vi "cam0-镜像槽点对应中心槽角计算.vi"(9 "位置参数":T1={"槽点位"={"X"=125.0, "Y"=75.0}, "产品位"={"X"=150.0, "Y"=100.0}, "各槽角"=[], "中心位"={"X"=100.0, "Y"=100.0}, "中心产品半径"=0.0, "最接近槽角序号"=0, "槽在中心到产品连线所在侧"=enum."左侧-逆时针向", "中心位到产品位指向角"=0.0}) -> (0 "匹配槽OK":bool, 2 "匹配到的槽角序号":i32, 3 "槽点偏距与产品半径比":dbl format="%.2f")   [LabVIEW 2018]
uses:
  <vilib>/vision/NI_Vision_Development_Module.lvlib
panel:
  # "槽点偏距与产品半径比，表示槽的对正程度，用于确定是否可以将该槽用于铜碎检测"
  # "反映了槽偏离中心线的程度"
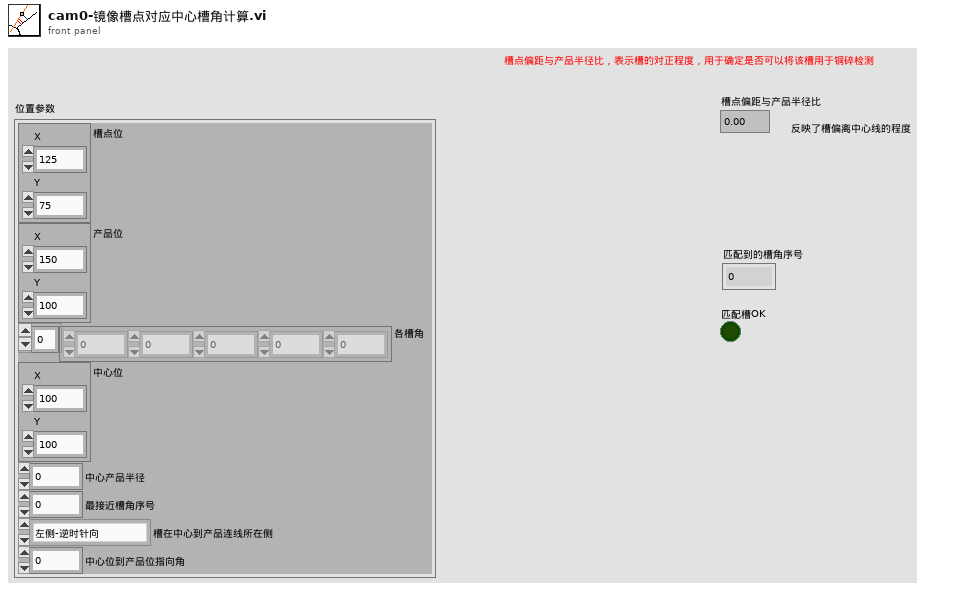
[diagram p1: front panel]
types:
  T1 = cluster{"槽点位":cluster{"X":sgl, "Y":sgl}, "产品位":cluster{"X":sgl, "Y":sgl}, "各槽角":dbl[], "中心位":cluster{"X":sgl, "Y":sgl}, "中心产品半径":sgl, "最接近槽角序号":i32, "槽在中心到产品连线所在侧":enum16{"左侧-逆时针向", "右侧-顺时针向"}, "中心位到产品位指向角":sgl}
  T2 = cluster{"产品位":cluster{"X":sgl, "Y":sgl}, "中心位":cluster{"X":sgl, "Y":sgl}}
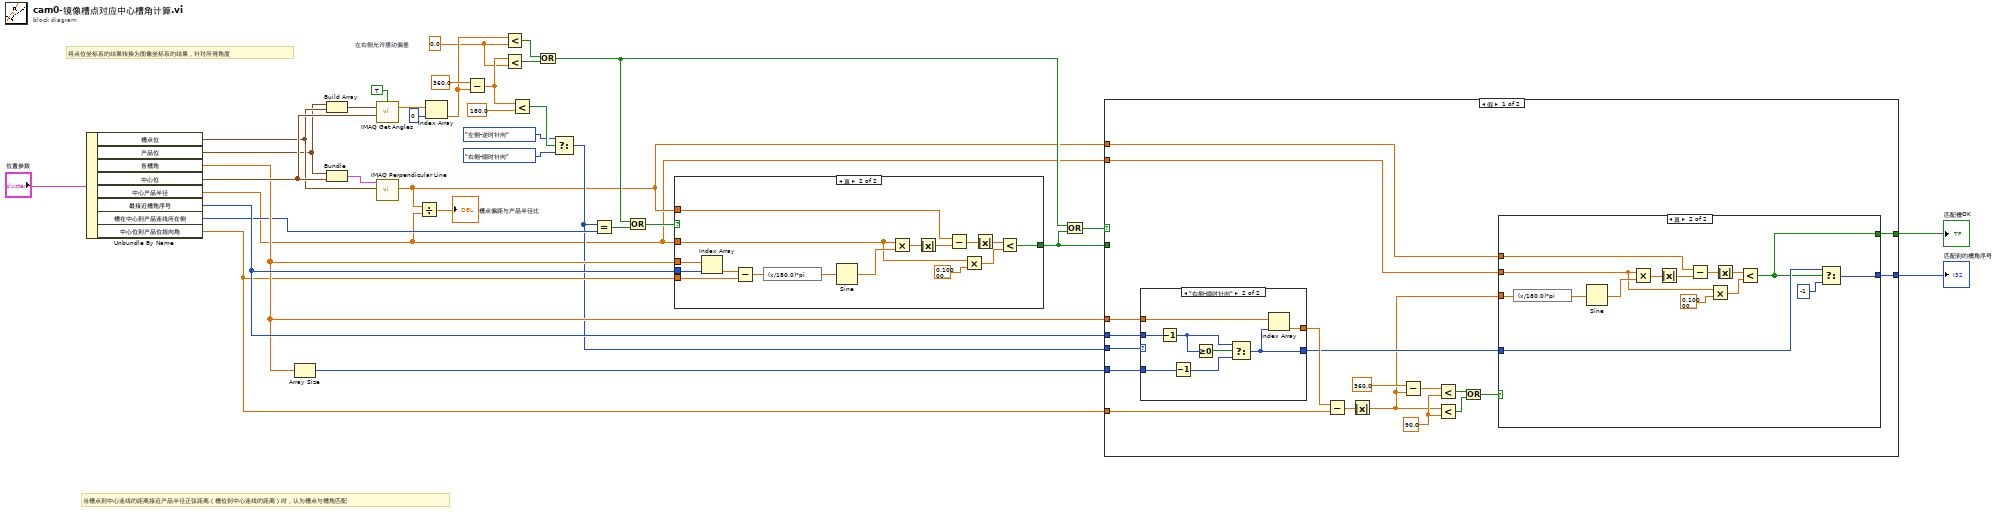
[diagram p0: block diagram]
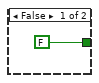
[diagram p2: hidden frame]
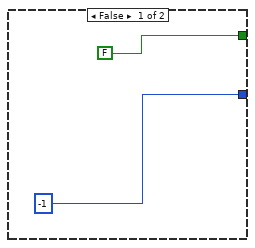
[diagram p3: hidden frame]
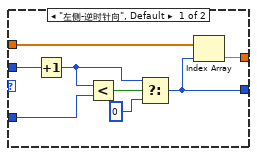
[diagram p4: hidden frame]
diagram:
  w11 = sgl 0.0  # 左右侧允许摆动偏差
  # "当槽点到中心连线的距离接近产品半径正弦距离（槽位到中心连线的距离）时，认为槽点与槽角匹配"
  # "将点位坐标系的结果转换为图像坐标系的结果，针对所得角度"
  n1 = Unbundle By Name("位置参数") -> ("槽点位"=w27:cluster{"X":sgl, "Y":sgl}, "产品位"=w26:cluster{"X":sgl, "Y":sgl}, "各槽角"=w22:dbl[], "中心位"=w28:cluster{"X":sgl, "Y":sgl}, "中心产品半径"=w2:sgl, "最接近槽角序号"=w24:i32, "槽在中心到产品连线所在侧"=w15:enum16{"左侧-逆时针向", "右侧-顺时针向"}, "中心位到产品位指向角"=w21:sgl)
  n2 = Array Size(array=w22) -> (size(s)=w23:i32)
  n3 = Build Array(w26, w27) -> (w31:cluster{"X":sgl, "Y":sgl}[])
  n4 = Bundle("产品位"=w26, "中心位"=w28) -> (w35:T2)  [unwired: 1 in]
  n5 = call "IMAQ Get Angles"("Vertex"=w28, "Points"=w31, "Use Vertex (No)"=TRUE) -> ("Angles (deg)"=w33:sgl[])  [unwired: 2 in, 2 out]
  n6 = call "IMAQ Perpendicular Line"("Point"=w27, "Line"=w35) -> ("Distance"=w3:dbl)  [unwired: 7 in, 2 out]
  n7 = Divide(x=w3, y=w2) -> (x/y=→"槽点偏距与产品半径比":dbl)
  n8 = Index Array(array=w33, index=0 ("索引")) -> (element=w12:sgl)
  n9 = Subtract(x=sgl 360.0, y=w12) -> (x-y=w13:sgl)
  n10 = Less?(x=w12, y=w11) -> (x < y?=w9:bool)
  n11 = Less?(x=w13, y=w11) -> (x < y?=w10:bool)
  n12 = Less?(x=w13, y=sgl 180.0) -> (x < y?=w18:bool)
  n13 = Or(x=w9, y=w10) -> (x .or. y?=w6:bool)
  n14 = Select(t=enum16{"左侧-逆时针向", "右侧-顺时针向"}."左侧-逆时针向" ("槽在中心到产品连线所在侧"), s=w18, f=enum16{"左侧-逆时针向", "右侧-顺时针向"}."右侧-顺时针向" ("槽在中心到产品连线所在侧")) -> (s? t:f=w14:enum16{"左侧-逆时针向", "右侧-顺时针向"})
  n15 = Equal?(x=w14, y=w15) -> (x = y?=w4:bool)
  n16 = Or(x=w6, y=w4) -> (x .or. y?=w5:bool)
  n17 = case shown="真" w5 {
    tunnel: [FALSE w44] -> w7
    tunnel: w24 -> [_ w43]
    tunnel: w22 -> [_ w42]
    tunnel: w21 -> [_ w41]
    tunnel: w3 -> [_ w39]
    tunnel: w2 -> [_ w37]
    frame False {
    }
    frame True {
      n18 = Index Array(array=w42, index=w43) -> (element=w45:dbl)
      n19 = Subtract(x=w45, y=w41) -> (x-y=w40:dbl)
      n20 = expression code="(x/180.0)*pi" ("degrees to radians")(w40) -> (w52:dbl)
      n21 = Sine(x=w52) -> (sin(x)=w51:dbl)
      n22 = Multiply(x=w37, y=w51) -> (x*y=w50:dbl)
      n23 = Absolute Value(x=w50) -> (abs(x)=w49:dbl)
      n24 = Subtract(x=w39, y=w49) -> (x-y=w48:dbl)
      n25 = Multiply(x=w37, y=sgl 0.1) -> (x*y=w38:sgl)
      n26 = Absolute Value(x=w48) -> (abs(x)=w47:dbl)
      n27 = Less?(x=w47, y=w38) -> (x < y?=w44:bool)
    }
  }
  n28 = Or(x=w6, y=w7) -> (x .or. y?=w8:bool)
  n29 = case shown="假" w8 {
    tunnel: [w57 w105] -> w25
    tunnel: w24 -> [w70 w106]
    tunnel: w14 -> [w71 _]
    tunnel: w23 -> [w69 _]
    tunnel: w22 -> [w68 _]
    tunnel: w21 -> [w66 _]
    tunnel: w3 -> [w56 _]
    tunnel: [w58 w106] -> w20
    tunnel: w2 -> [w55 _]
    tunnel: w7 -> [_ w105]
    frame False {
      w63 = 90.0 ("y")
      n30 = case shown="\"右侧-顺时针向\"" w71 {
        tunnel: w70 -> [w96 w102]
        tunnel: w69 -> [w95 w100]
        tunnel: w68 -> [w91 w103]
        tunnel: [w90 w98] -> w67
        tunnel: [w89 w97] -> w59
        frame "左侧-逆时针向", Default {
          n31 = Increment(x=w96) -> (x+1=w93:i32)
          n32 = Less?(x=w93, y=w95) -> (x < y?=w94:bool)
          n33 = Select(t=w93, s=w94, f=0) -> (s? t:f=w89:i32)
          n34 = Index Array(array=w91, index=w89) -> (element=w90:dbl)
        }
        frame "右侧-顺时针向" {
          n35 = Decrement(x=w102) -> (x-1=w101:i32)
          n36 = Decrement(x=w100) -> (x-1=w99:i32)
          n37 = Greater Or Equal To 0?(x=w101) -> (x >= 0?=w104:bool)
          n38 = Select(t=w101, s=w104, f=w99) -> (s? t:f=w97:i32)
          n39 = Index Array(array=w103, index=w97) -> (element=w98:dbl)
        }
      }
      n40 = Subtract(x=w67, y=w66) -> (x-y=w54:dbl)
      n41 = Absolute Value(x=w54) -> (abs(x)=w53:dbl)
      n42 = Subtract(x=360.0, y=w53) -> (x-y=w64:dbl)
      n43 = Less?(x=w64, y=w63) -> (x < y?=w62:bool)
      n44 = Less?(x=w53, y=w63) -> (x < y?=w61:bool)
      n45 = Or(x=w62, y=w61) -> (x .or. y?=w60:bool)
      n46 = case shown="真" w60 {
        tunnel: w53 -> [_ w87]
        tunnel: w55 -> [_ w74]
        tunnel: w59 -> [_ w81]
        tunnel: [-1 ("f") w79] -> w58
        tunnel: [FALSE w78] -> w57
        tunnel: w56 -> [_ w77]
        frame False {
        }
        frame True {
          n47 = expression code="(x/180.0)*pi" ("degrees to radians")(w87) -> (w88:dbl)
          n48 = Sine(x=w88) -> (sin(x)=w82:dbl)
          n49 = Multiply(x=w74, y=w82) -> (x*y=w83:dbl)
          n50 = Absolute Value(x=w83) -> (abs(x)=w84:dbl)
          n51 = Subtract(x=w77, y=w84) -> (x-y=w85:dbl)
          n52 = Multiply(x=w74, y=sgl 0.1) -> (x*y=w75:sgl)
          n53 = Absolute Value(x=w85) -> (abs(x)=w86:dbl)
          n54 = Less?(x=w86, y=w75) -> (x < y?=w78:bool)
          n55 = Select(t=w81, s=w78, f=-1) -> (s? t:f=w79:i32)
        }
      }
    }
    frame True {
    }
  }
  "匹配槽OK" <- w25
  "匹配到的槽角序号" <- w20
